vi "rx.vi"(8 "error in (no error)":errorcluster, 11 "tcp server in":refnum<class "tcp connection.lvclass">) -> (0 "error out":errorcluster, 1 "new message":bool, 2 "rx":string, 3 "tcp server out":refnum<class "tcp connection.lvclass">)   [LabVIEW 2014, in "tcp connection.lvclass"]
uses:
  tcp connection.lvclass
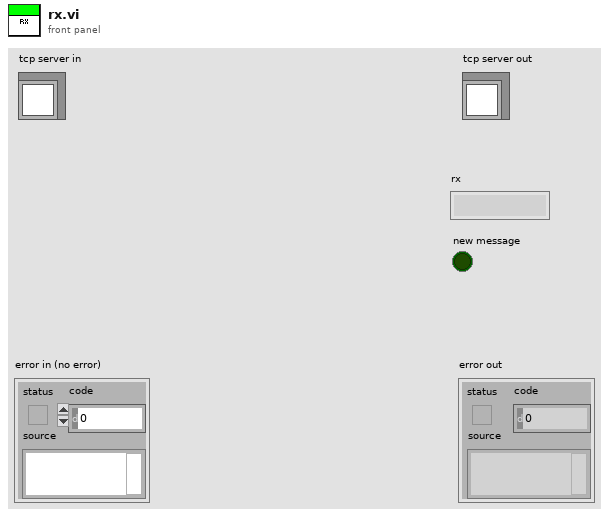
[diagram p1: front panel]
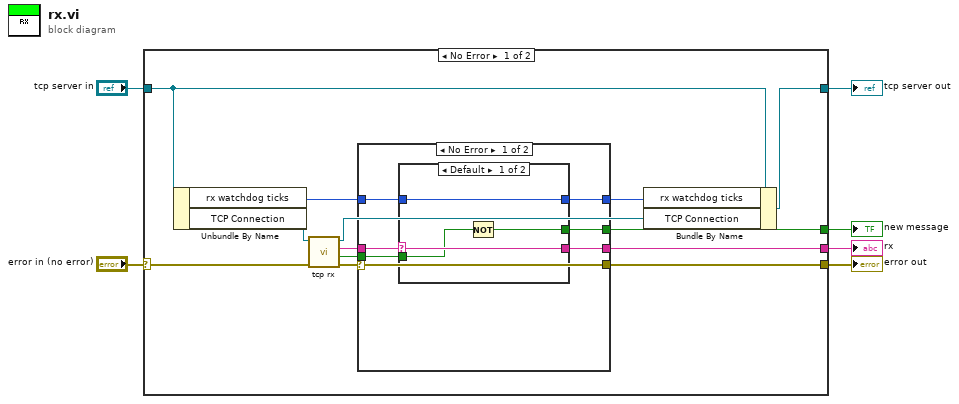
[diagram p0: block diagram]
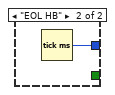
[diagram p2: hidden frame]
diagram:
  n1 = case shown="No Error" "error in (no error)" {
    selector: "error in (no error)" -> [w14 w35]
    tunnel: [w19 w35] -> w5
    tunnel: [w17 w34] -> w3
    tunnel: "tcp server in" -> [w18 w34]
    tunnel: [w10 _] -> w2
    tunnel: [w7 _] -> w1
    frame No Error {
      n2 = Unbundle By Name(w18) -> ("rx watchdog ticks"=w16:u32, "TCP Connection"=w12:refnum<k5>)
      n3 = call "tcp rx.vi"("error in"=w14, "TCP Connection in"=w12) -> ("error out"=w13:errorcluster, "poll timeout"=w8:bool, "rx"=w11:string, "TCP Connection out"=w9:refnum<k5>)  [unwired: 6 in]
      n4 = case shown="No Error" w13 {
        selector: w13 -> [w26 w32]
        tunnel: [w26 w32] -> w19
        tunnel: w16 -> [w24 w33]
        tunnel: [w25 w33] -> w15
        tunnel: w11 -> [w23 _]
        tunnel: [w22 _] -> w10
        tunnel: w8 -> [w21 _]
        tunnel: [w20 _] -> w7
        frame No Error {
          n5 = case shown="Default" w23 {
            selector: w23 -> [w30 _]
            tunnel: [w30 _] -> w22
            tunnel: [w29 w31] -> w25
            tunnel: w24 -> [w29 _]
            tunnel: w21 -> [w28 _]
            tunnel: [w27 _] -> w20
            frame Default {
              n6 = Not(x=w28) -> (.not. x?=w27:bool)
            }
            frame "EOL HB" {
              n7 = Tick Count (ms)() -> (millisecond timer value=w31:u32)
            }
          }
        }
        frame Error {
        }
      }
      n8 = Bundle By Name(cluster=w18, "rx watchdog ticks"=w15, "TCP Connection"=w9) -> (w17:refnum<class "tcp connection.lvclass">)
    }
    frame Error {
    }
  }
  "error out" <- w5
  "tcp server out" <- w3
  "rx" <- w2
  "new message" <- w1
